vi "Get Resource Type.vi"(11 "GPIO in":refnum<class "GPIO.lvclass">) -> (2 "Resource Type":string)   [LabVIEW 2020, in "CTI.lvlib" / "GPIO.lvclass"]
uses:
  GPIO.lvclass
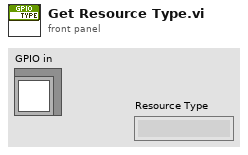
[diagram p1: front panel]
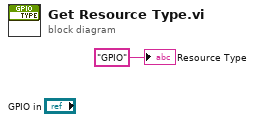
[diagram p0: block diagram]
diagram:
  "Resource Type" <- "GPIO" ("Resource Type")
